vi "SS_FPGA_Drop1_all_in_v4.vi"() -> ()   [LabVIEW 2016]
uses:
  <vilib>/rvi/Emulation/niFpgaGetClockAttributes.vi
  <vilib>/rvi/Emulation/niFpgaSctlEmulationGetInTimedLoop.vi
  <vilib>/rvi/Emulation/niFpgaEmulationReportErrorSimple.vi
  <vilib>/rvi/Emulation/niFpgaCriticalErrorInLSC.vi
  <vilib>/rvi/Emulation/niFpgaProcessEmulError.vi
  <vilib>/rvi/eio/common/nirviEmuTemplateMethod_errors.vi
  <vilib>/eio/EIONode/EIONode.xnode
  <vilib>/rvi/FXPMathLib/FxpMul/XNode/nifxpmath_Multiplier.xnode
  <vilib>/rvi/FXPMathLib/FxpAdd/XNode/nifxpmath_Add.xnode
  <vilib>/rvi/FXPMathLib/sim/FxpSim.dll
panel:
  in  "Tab Control":T1(tab)
  in  "(FOR DEBUG) Overide FBIS 1kHZ":bool
  in  "Start Acquisition":bool
  out "Actual Duration (ms)":u32
  out "Number of Loop 1 Samples":i32
  in  "Scan Rate (mSec) Loop 1":u32 caption="Count(mSec)"
  in  "FSIS Interlock":bool
  out "Raw Data In Mod 1":fxp<+,24,12>[](array[numeric])
  out "Cal value out Mod 1":fxp<+,24,12>[](array[numeric]) format="%.16g"
  out "PTF - No Operations Mod 1":bool[](array[boolean])
  in  "lower limit \nNOOP mod 1":fxp<+,24,12>[](array[numeric])=[0.0, 0.0, 0.0, 0.0, 0.0, 0.0, 0.0, 0.0, 0.0, 0.0, 0.0, 0.0, 0.0, 0.0, 0.0, 0.0]
  in  "upper limit \nOKOP mod 1":fxp<+,24,12>[](array[numeric])=[0.0, 0.0, 0.0, 0.0, 0.0, 0.0, 0.0, 0.0, 0.0, 0.0, 0.0, 0.0, 0.0, 0.0, 0.0, 0.0]
  out "PTF - Warning Mod 1":bool[](array[boolean])
  in  "NOOPS Fault Filter mod 1":u16[](array[numeric])=[0, 0, 0, 0, 0, 0, 0, 0, 0, 0, 0, 0, 0, 0, 0, 0]
  in  "cal mod 1":fxp<+,24,12>[](array[numeric])=[10.0, 10.0, 10.0, 10.0, 10.0, 10.0, 10.0, 10.0, 10.0, 10.0, 10.0, 10.0, 10.0, 10.0, 10.0, 10.0]
  in  "offset mod 1":fxp<+,24,12>[](array[numeric])=[0.0, 0.0, 0.0, 0.0, 0.0, 0.0, 0.0, 0.0, 0.0, 0.0, 0.0, 0.0, 0.0, 0.0, 0.0, 0.0]
  out "Raw Data In Mod 2":fxp<+,24,12>[](array[numeric]) format="%.27g"
  in  "offset mod 2":fxp<+,24,12>[](array[numeric])=[0.0, 0.0, 0.0, 0.0, 0.0, 0.0, 0.0, 0.0, 0.0, 0.0, 0.0, 0.0, 0.0, 0.0, 0.0, 0.0]
  out "PTF - No Operations Mod 2":bool[](array[boolean])
  in  "lower limit \nNOOP mod 2":fxp<+,24,12>[](array[numeric])=[0.0, 0.0, 0.0, 0.0, 0.0, 0.0, 0.0, 0.0, 0.0, 0.0, 0.0, 0.0, 0.0, 0.0, 0.0, 0.0]
  in  "upper limit \nOKOP mod 2":fxp<+,24,12>[](array[numeric])=[0.0, 0.0, 0.0, 0.0, 0.0, 0.0, 0.0, 0.0, 0.0, 0.0, 0.0, 0.0, 0.0, 0.0, 0.0, 0.0]
  out "Cal value out Mod 2":fxp<+,24,12>[](array[numeric])
  out "PTF - Warning Mod 2":bool[](array[boolean])
  in  "NOOPS Fault Filter mod 2":u16[](array[numeric])=[0, 0, 0, 0, 0, 0, 0, 0, 0, 0, 0, 0, 0, 0, 0, 0]
  in  "cal mod 2":fxp<+,24,12>[](array[numeric])=[0.0, 0.0, 0.0, 0.0, 0.0, 0.0, 0.0, 0.0, 0.0, 0.0, 0.0, 0.0, 0.0, 0.0, 0.0, 0.0]
  out "Raw Data In Mod 3":fxp<+,24,12>[](array[numeric]) format="%.27g"
  out "PTF - No Operations Mod 3":bool[](array[boolean])
  in  "lower limit\nNOOP mod 3":fxp<+,24,12>[](array[numeric])=[0.0, 0.0, 0.0, 0.0, 0.0, 0.0, 0.0, 0.0, 0.0, 0.0, 0.0, 0.0, 0.0, 0.0, 0.0, 0.0]
  in  "upper limit\nOKOP mod 3":fxp<+,24,12>[](array[numeric])=[0.0, 0.0, 0.0, 0.0, 0.0, 0.0, 0.0, 0.0, 0.0, 0.0, 0.0, 0.0, 0.0, 0.0, 0.0, 0.0]
  out "PTF - Warning Mod 3":bool[](array[boolean])
  out "Cal value out Mod 3":fxp<+,24,12>[](array[numeric])
  in  "NOOPS Fault Filter mod 3":u16[](array[numeric])=[0, 0, 0, 0, 0, 0, 0, 0, 0, 0, 0, 0, 0, 0, 0, 0]
  in  "offset mod 3":fxp<+,24,12>[](array[numeric])=[0.0, 0.0, 0.0, 0.0, 0.0, 0.0, 0.0, 0.0, 0.0, 0.0, 0.0, 0.0, 0.0, 0.0, 0.0, 0.0]
  in  "cal mod 3":fxp<+,24,12>[](array[numeric])=[0.0, 0.0, 0.0, 0.0, 0.0, 0.0, 0.0, 0.0, 0.0, 0.0, 0.0, 0.0, 0.0, 0.0, 0.0, 0.0]
  out "Raw Data In Mod 4":fxp<+,24,12>[](array[numeric]) format="%.27g"
  out "Cal value out Mod 4":fxp<+,24,12>[](array[numeric])
  out "PTF - No Operations Mod 4":bool[](array[boolean])
  out "PTF - Warning Mod 4":bool[](array[boolean])
  in  "lower limit\nNOOP mod 4":fxp<+,24,12>[](array[numeric])=[0.0, 0.0, 0.0]
  in  "upper limit\nOKOP mod 4":fxp<+,24,12>[](array[numeric])=[0.0, 0.0, 0.0]
  in  "cal mod 4":fxp<+,24,12>[](array[numeric])=[0.0, 0.0, 0.0]
  in  "NOOPS Fault Filter mod 4":u16[](array[numeric])=[0, 0, 0]
  in  "offset mod 4":fxp<+,24,12>[](array[numeric])=[0.0, 0.0, 0.0]
  out "Cal value out Mod 5":fxp<+,24,12>[](array[numeric])
  out "PTF - No Operations Mod 5":bool[](array[boolean])
  out "PTF - Warning Mod 5":bool[](array[boolean])
  in  "lower limit\nNOOP mod 5":fxp<+,24,12>[](array[numeric])=[0.0, 0.0, 0.0]
  in  "upper limit\nOKOP mod 5":fxp<+,24,12>[](array[numeric])=[0.0, 0.0, 0.0]
  in  "cal mod 5":fxp<+,24,12>[](array[numeric])=[0.0, 0.0, 0.0]
  in  "NOOPS Fault Filter mod 5":u16[](array[numeric])=[0, 0, 0]
  in  "offset mod 5":fxp<+,24,12>[](array[numeric])=[0.0, 0.0, 0.0]
  out "Raw Data In Mod 5":fxp<+,24,12>[](array[numeric]) format="%.27g"
  out "Raw Data In Mod 6":bool[](array[boolean])
  out "Trigger from Trigger Card (SYNC and ASYNC) (Euro1Slot15)":bool
  out "Main Trigger In":bool
  out "SYNC/ASYNC":bool
  out "Beam Prepare":bool
  out "Override":bool
  out "320 Open":bool
  out "320  Closed":bool
  out "400 Open":bool
  out "400 Open Closed":bool
  out "Calorimeter Left Gate Open":bool
  out "Calorimeter Left Gate Closed":bool
  out "320  Bypass Open":bool
  out "320 Bypass Closed":bool
  out "Calorimeter Right Gate Closed":bool
  out "HV Area Water":bool
  out "MAST Area Air":bool
  out "Calorimeter Right Gate Open":bool
  # "1"
  # "2"
  # "CHANNEL ID"
  # "SS Source Body Flow\n\nSS Source Body Temperature\n\nSS Grid 1 Flow\n\nSS Grid 1 Temperature\n\nSS Grid 2 Flow\n\nSS Grid 2 Temperature\n\nSS Grid 3 Flow\n\nSS Grid 3 Temperature\n\nSS Grid 4/1st Stage Neutraliser Flow\n\nSS Grid 4/1st Stage Neutraliser Temperature\n\nSS 2nd Stage Neutraliser Flow\n\nSS 2nd Stage Neutraliser Temperature\n\nSS PINI Backplate Flow\n\nSS PINI Backplate Temperature\n\nSS Duct Scraper Flow\n\nSS Duct Scraper Temperature"
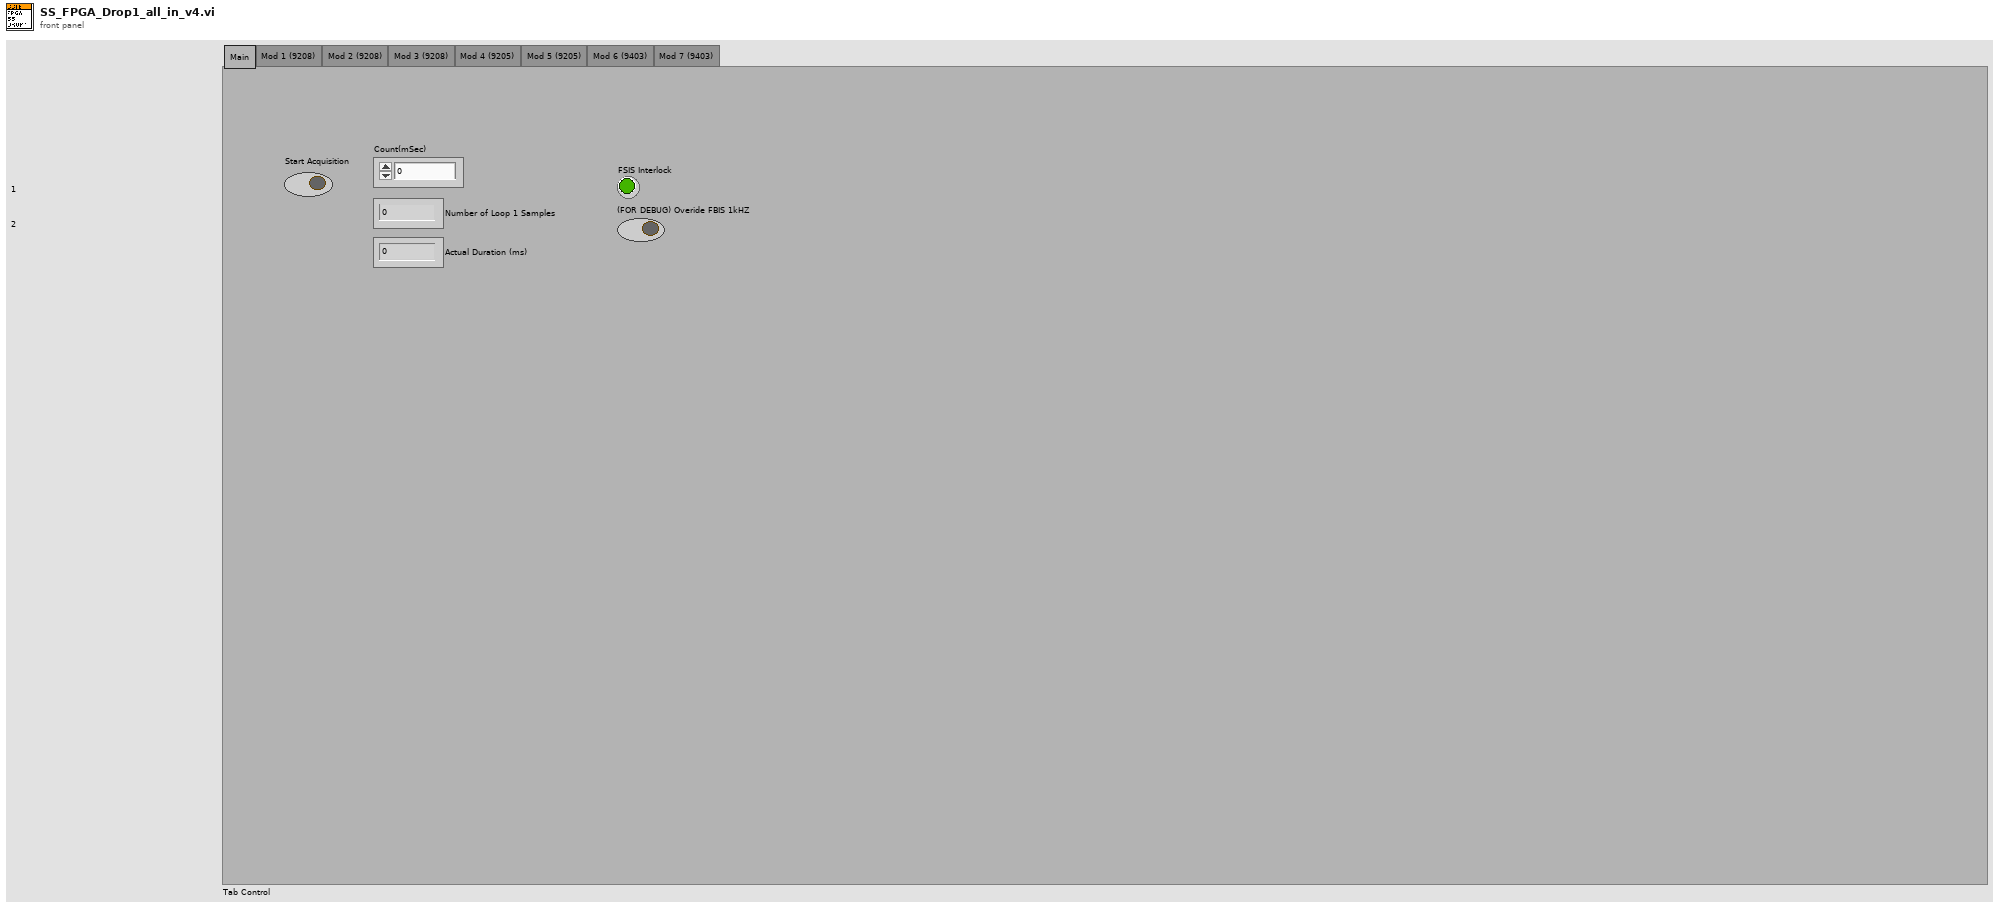
[diagram p1: front panel]
types:
  T1 = enum32{"Main", "Mod 1 (9208)", "Mod 2 (9208)", "Mod 3 (9208)", "Mod 4 (9205)", "Mod 5 (9205)", "Mod 6 (9403)", "Mod 7 (9403)"}
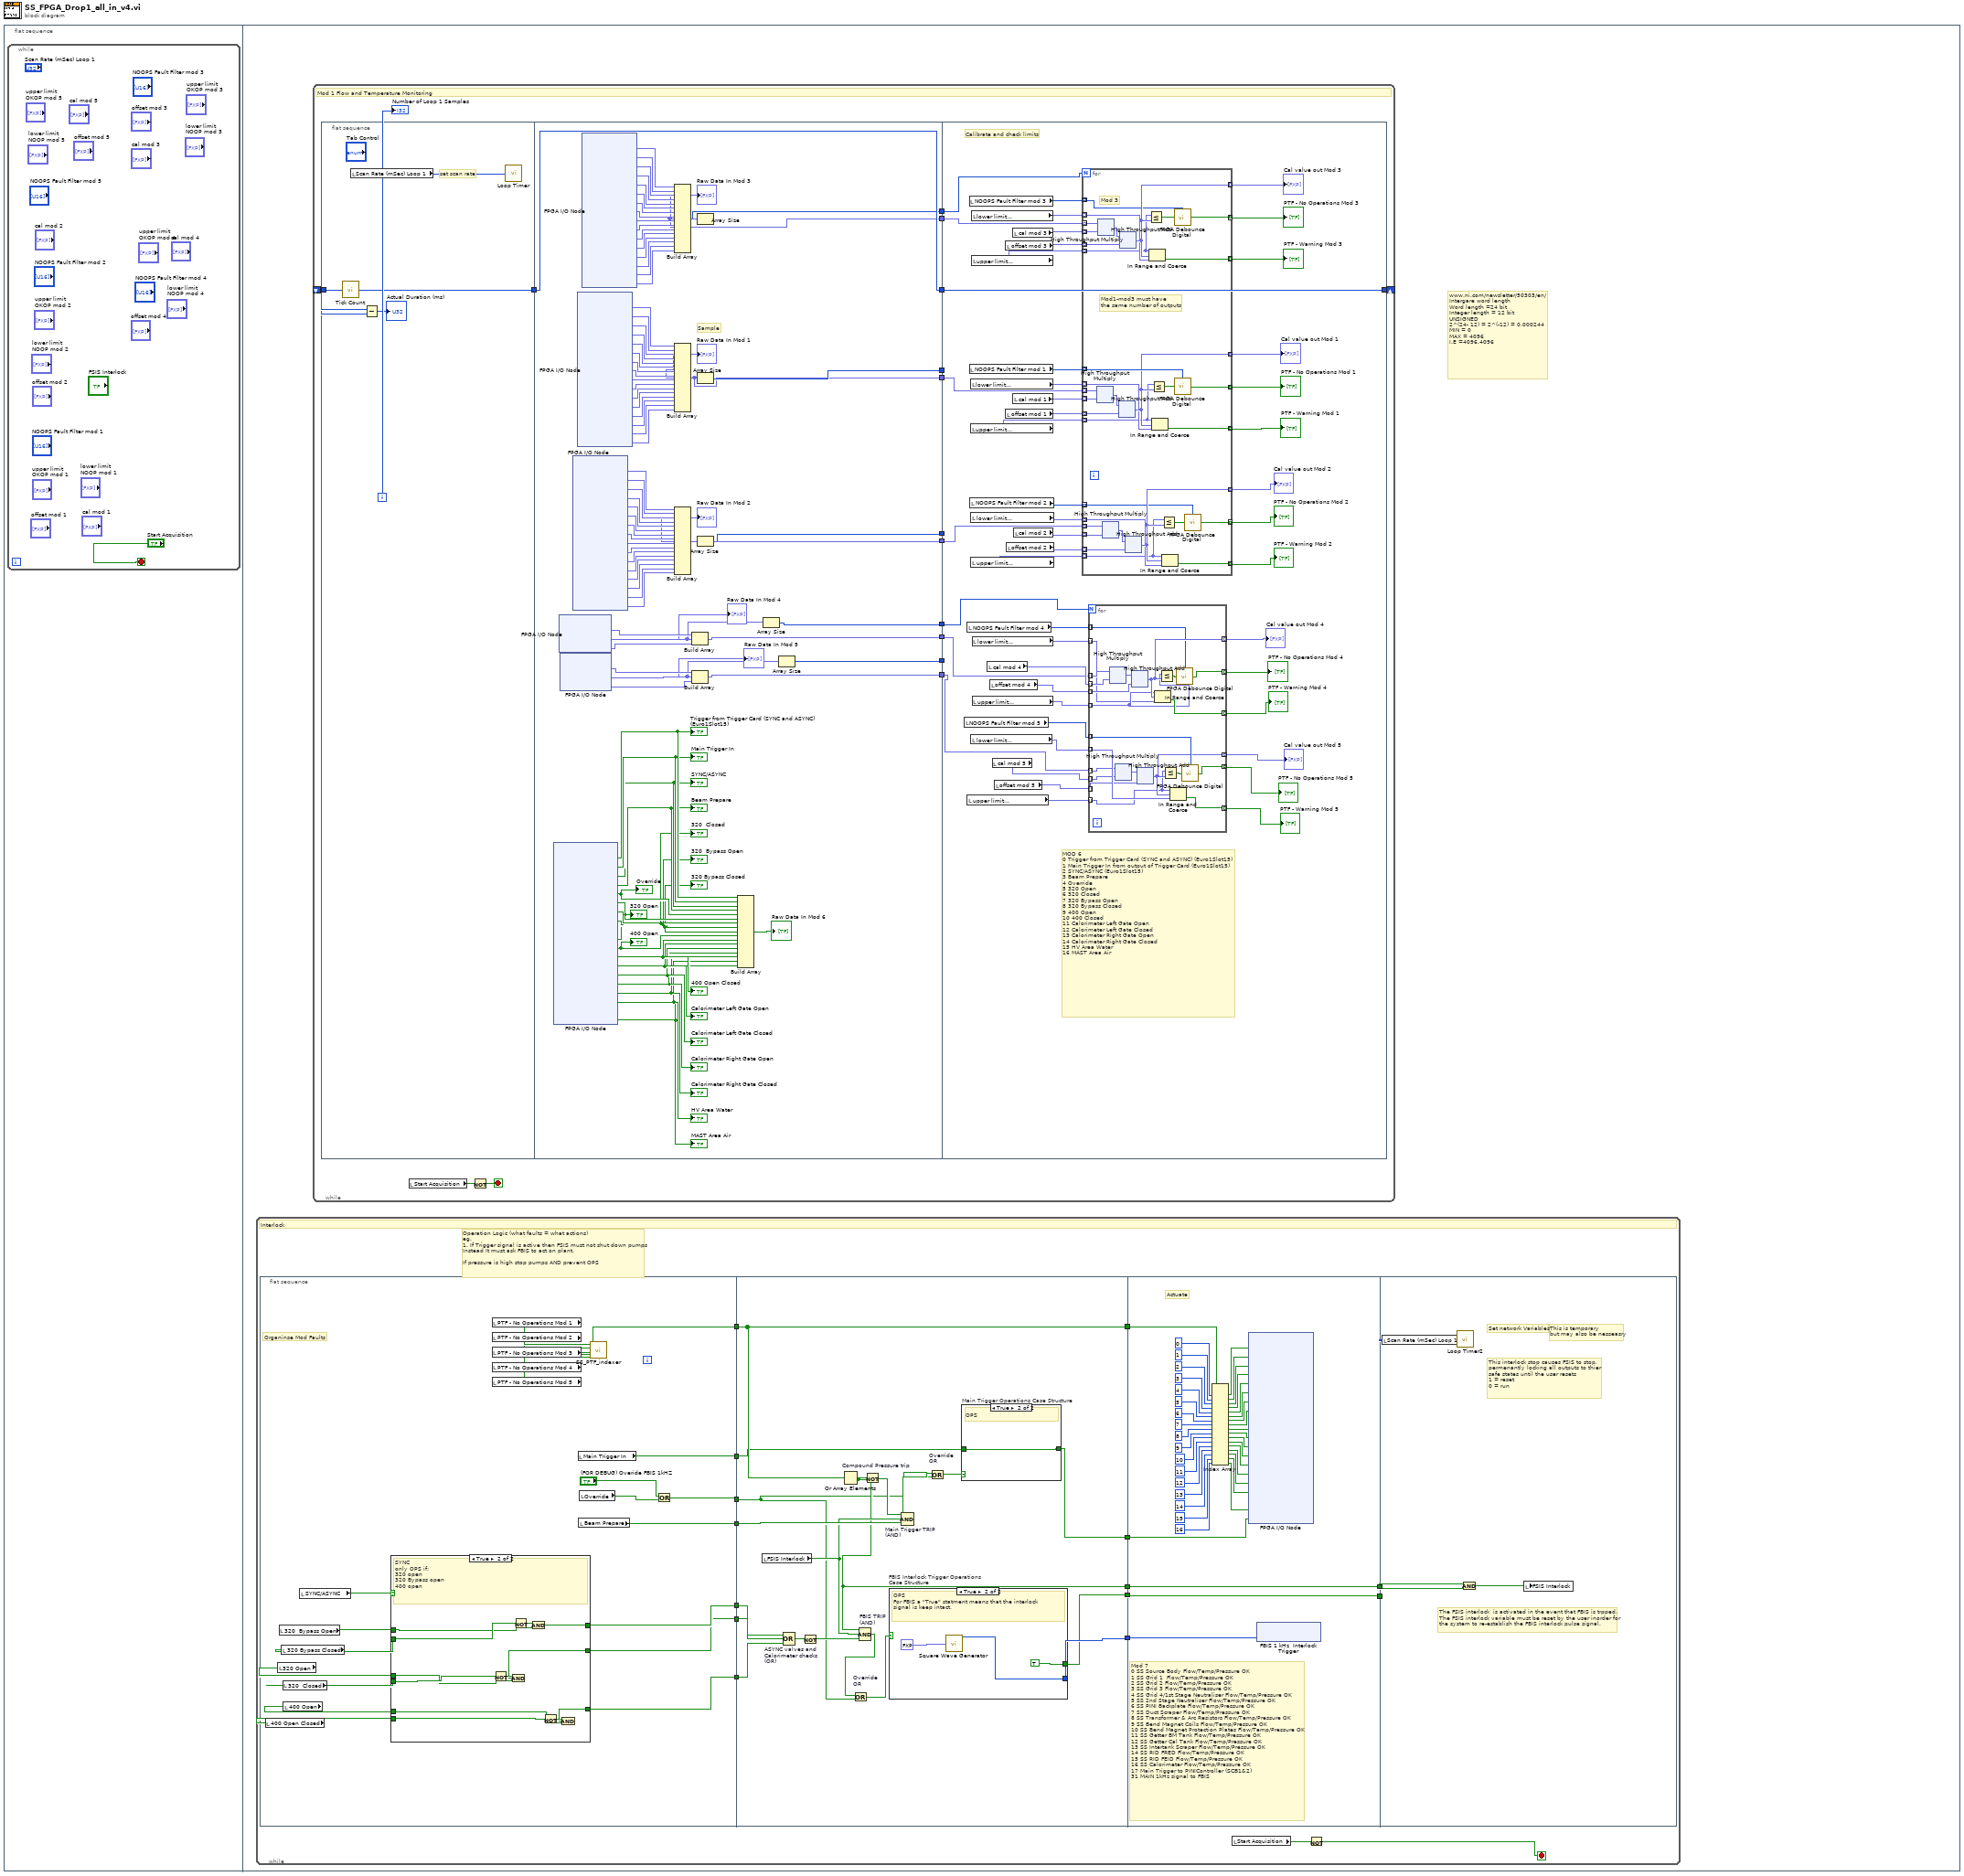
[diagram p0: block diagram]
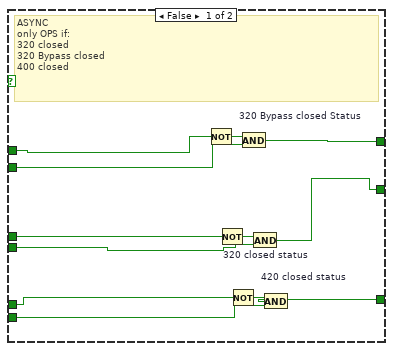
[diagram p2: hidden frame]
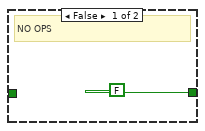
[diagram p3: hidden frame]
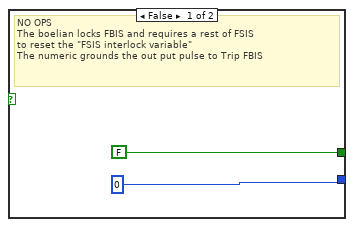
[diagram p4: hidden frame]
diagram:
  n1 = flat-sequence {
    frame #0 {
      n2 = while {
        stop <- "Start Acquisition" stop-if-true
      }
    }
    frame #1 {
      # "www.ni.com/newsletter/50303/en/\nIntergare word length \nWord length =24 bit\nInteger length = 12 bit\nUNSIGNED\n2^(24- 12) = 2^(-12) = 0.000244\nMIN = 0 \nMAX = 4096\nI.E =4096.4096"
      n3 = while {
        stop <- w8 stop-if-true
        # "Operation Logic (what faults = what actions)\neg.\n1. If Trigger signal is active then FSIS must not shut down pumps\nInstead It must ask FBIS to act on plant.\n\nIf pressure is high stop pumps AND prevent OPS"
        # "Interlock"
        n4 = flat-sequence {
          tunnel: [w32] -> w17
          tunnel: [w31] -> w16
          tunnel: [w30] -> w15
          tunnel: [w29] -> w13
          tunnel: [w24] -> w10
          tunnel: [w21] -> w3
          tunnel: [w20] -> w2
          tunnel: w17 -> [w75]
          tunnel: w16 -> [w74]
          tunnel: w15 -> [w73]
          tunnel: [w81] -> w14
          tunnel: w13 -> [w79]
          tunnel: [w68] -> w12
          tunnel: w10 -> [w80]
          tunnel: [w80] -> w9
          tunnel: [w78] -> w6
          tunnel: [w77] -> w5
          tunnel: w3 -> [w70]
          tunnel: w2 -> [w63]
          tunnel: w14 -> [w127]
          tunnel: w12 -> [w126]
          tunnel: [w126] -> w11
          tunnel: w9 -> [w125]
          tunnel: w6 -> [w90]
          tunnel: w5 -> [w89]
          tunnel: [w89] -> w4
          tunnel: w11 -> [w129]
          tunnel: w4 -> [w128]
          frame #0 {
            # "Organinse Mod Faults"
            n5 = local read "400 Open Closed"() -> (w35:bool)
            n6 = local read "320 Open"() -> (w33:bool)
            n7 = local read "320  Bypass Open"() -> (w37:bool)
            n8 = local read "320 Bypass Closed"() -> (w34:bool)
            n9 = local read "320  Closed"() -> (w22:bool)
            n10 = local read "400 Open"() -> (w36:bool)
            n11 = local read "SYNC/ASYNC"() -> (w38:bool)
            n12 = case shown="True" w38 {
              tunnel: w37 -> [w50 w58]
              tunnel: w36 -> [w42 w56]
              tunnel: w35 -> [w46 w57]
              tunnel: w34 -> [w45 w59]
              tunnel: w22 -> [w44 w55]
              tunnel: w33 -> [w43 w54]
              tunnel: [w39 w51] -> w30
              tunnel: [w41 w52] -> w31
              tunnel: [w40 w53] -> w32
              frame False {
                # "ASYNC\nonly OPS if:\n320 closed\n320 Bypass closed\n400 closed"
                n13 = Not(x=w50) -> (.not. x?=w49:bool)
                n14 = Not(x=w43) -> (.not. x?=w48:bool)
                n15 = Not(x=w42) -> (.not. x?=w47:bool)
                n16 = And "320 Bypass closed Status"(x=w49, y=w45) -> (x .and. y?=w40:bool)
                n17 = And "320 closed status"(x=w48, y=w44) -> (x .and. y?=w41:bool)
                n18 = And "420 closed status"(x=w47, y=w46) -> (x .and. y?=w39:bool)
              }
              frame True {
                # "SYNC\nonly OPS if:\n320 open\n320 Bypass open\n400 open"
                n19 = Not(x=w55) -> (.not. x?=w60:bool)
                n20 = And(x=w60, y=w54) -> (x .and. y?=w52:bool)
                n21 = Not(x=w59) -> (.not. x?=w62:bool)
                n22 = And(x=w62, y=w58) -> (x .and. y?=w53:bool)
                n23 = Not(x=w57) -> (.not. x?=w61:bool)
                n24 = And(x=w61, y=w56) -> (x .and. y?=w51:bool)
              }
            }
            n25 = local read "PTF - No Operations Mod 1"() -> (w28:bool[])
            n26 = local read "PTF - No Operations Mod 2"() -> (w27:bool[])
            n27 = local read "PTF - No Operations Mod 3"() -> (w26:bool[])
            n28 = local read "PTF - No Operations Mod 4"() -> (w25:bool[])
            n29 = local read "PTF - No Operations Mod 5"() -> (w23:bool[])
            n30 = local read "Main Trigger In"() -> (w29:bool)
            n31 = local read "Beam Prepare"() -> (w21:bool)
            n32 = local read "Override"() -> (w18:bool)
            n33 = call "SS_PTF_indexer.vi"("Faults Mod 5"=w23, "Faults Mod 4"=w25, "Faults Mod 3"=w26, "Faults Mod 2"=w27, "Faults Mod 1"=w28) -> ("Group PTF"=w24:bool[])  [unwired: 6 in]
            n34 = Or(x="(FOR DEBUG) Overide FBIS 1kHZ", y=w18) -> (x .or. y?=w20:bool)
          }
          frame #1 {
            n35 = local read "FSIS Interlock"() -> (w69:bool)
            n36 = Compound Arithmetic op=OR "ASYNC valves and \nCalorimeter checks\n(OR)"(w75, w74, w73) -> (w72:bool)
            n37 = Not(x=w72) -> (.not. x?=w71:bool)
            n38 = Or Array Elements "Compound Pressure trip"(Boolean array=w80) -> (logical OR=w76:bool)
            n39 = Not(x=w76) -> (.not. x?=w68:bool)
            n40 = Compound Arithmetic op=AND "FBIS TRIP\n(AND)"(w68, w69, w71) -> (w67:bool)
            n41 = Or "Override \nOR"(x=w67, y=w63) -> (x .or. y?=w66:bool)
            n42 = case "FBIS Interlock Trigger Operations \nCase Structure" shown="True" w66 {
              tunnel: [u8 0 ("duty cycle (periods)") w87] -> w81
              tunnel: [FALSE TRUE] -> w77
              frame False {
                # "NO OPS\nThe boelian locks FBIS and requires a rest of FSIS \nto reset the \"FSIS interlock variable\"\nThe numeric grounds the out put pulse to Trip FBIS"
              }
              frame True {
                # "OPS\nFor FBIS a \"True\" statment means that the interlock\nsignal is keep intact."
                n43 = call "Square Wave Generator"("duty cycle (periods)"=fxp<+,32,0> 0.5) -> ("square wave out"=w87:i16)  [unwired: 14 in]
              }
            }
            n44 = Compound Arithmetic op=AND "Main Trigger TRIP\n(AND)"(w68, w69, w70) -> (w64:bool)
            n45 = Or "Override \nOR"(x=w64, y=w63) -> (x .or. y?=w65:bool)
            n46 = case "Main Trigger Operations Case Structure" shown="True" w65 {
              tunnel: w79 -> [_ w83]
              tunnel: [FALSE w83] -> w78
              frame False {
                # "NO OPS"
              }
              frame True {
                # "OPS"
              }
            }
          }
          frame #2 {
            # "Mod 7\n0\tSS Source Body Flow/Temp/Pressure OK\n1\tSS Grid 1  Flow/Temp/Pressure OK\n2\tSS Grid 2 Flow/Temp/Pressure OK\n3\tSS Grid 3 Flow/Temp/Pressure OK\n4\tSS Grid 4/1st Stage Neutraliser Flow/Temp/Pressure OK\n5\tSS 2nd Stage Neutraliser Flow/Temp/Pressure OK\n6\tSS PINI Backplate Flow/Temp/Pressure OK\n7\tSS Duct Scraper Flow/Temp/Pressure OK\n8\tSS Transformer & Arc Resistors Flow/Temp/Pressure OK\n9\tSS Bend Magnet Coils Flow/Temp/Pressure OK\n10\tSS Bend Magnet Protection Plates Flow/Temp/Pressure OK\n11\tSS Getter BM Tank Flow/Temp/Pressure OK\n12\tSS Getter Cal Tank Flow/Temp/Pressure OK\n13\tSS Intertank Scraper Flow/Temp/Pressure OK\n14\tSS RID FRED Flow/Temp/Pressure OK\n15\tSS RID FEID Flow/Temp/Pressure OK\n16\tSS Calorimeter Flow/Temp/Pressure OK\n17\tMain Trigger to PINIController (SCB1&2)\n31\tMAIN 1kHz signal to FBIS"
            # "Actuate"
            n47 = Index Array(array=w125, index #1=0 ("index"), index #2=1 ("index"), index #3=2 ("index"), index #4=3 ("index"), index #5=4 ("index"), index #6=5 ("index"), index #7=6 ("index"), index #8=7 ("index"), index #9=8 ("index"), index #10=9 ("index"), index #11=10 ("index"), index #12=11 ("index"), index #13=12 ("index"), index #14=13 ("index"), index #15=14 ("index"), index #16=15 ("index"), index #17=16 ("index")) -> (element #1=w108:bool, element #2=w107:bool, element #3=w106:bool, element #4=w105:bool, element #5=w104:bool, element #6=w103:bool, element #7=w102:bool, element #8=w101:bool, element #9=w100:bool, element #10=w99:bool, element #11=w98:bool, element #12=w97:bool, element #13=w96:bool, element #14=w95:bool, element #15=w93:bool, element #16=w92:bool, element #17=w91:bool)
            n48 = xnode "FPGA I/O Node"("Mod7/DIO0"=w108, "Mod7/DIO1"=w107, "Mod7/DIO2"=w106, "Mod7/DIO3"=w105, "Mod7/DIO4"=w104, "Mod7/DIO5"=w103, "Mod7/DIO6"=w102, "Mod7/DIO7"=w101, "Mod7/DIO8"=w100, "Mod7/DIO9"=w99, "Mod7/DIO10"=w98, "Mod7/DIO11"=w97, "Mod7/DIO12"=w96, "Mod7/DIO13"=w95, "Mod7/DIO14"=w93, "Mod7/DIO15"=w92, "Mod7/DIO16"=w91, "Mod7/DIO17"=w90) -> ()  [unwired: 20 in, 22 out]
            n49 = xnode "FBIS 1 kHz  Interlock Trigger"("Mod7/DIO31:0"=w127) -> ()  [unwired: 1 in, 1 out]
          }
          frame #3 {
            # "The FSIS interlock  is activated in the event that FBIS is trpped.\nThe FSIS interlock variable must be reset by the user inorder for \nthe system to re-establish the FBIS interlock pulse signal."
            # "This interlock stop causes FSIS to stop,\npermenantly locking all outputs to thier \nsafe states until the user resets\n1 = reset\n0 = run"
            # "This is temporary\nbut may also be nesseasry"
            # "Set network Variables"
            n50 = local read "Scan Rate (mSec) Loop 1"() -> (w131:u32)
            n51 = call "Loop Timer2"("Count(mSec)"=w131) -> ()  [unwired: 1 out]
            n52 = And(x=w129, y=w128) -> (x .and. y?=w130:bool)
            n53 = local write "FSIS Interlock"(w130) -> ()
          }
        }
        n54 = local read "Start Acquisition"() -> (w7:bool)
        n55 = Not(x=w7) -> (.not. x?=w8:bool)
      }
      n56 = while {
        shift-right: [w147] -> _
        shift-left: _ -> [w145]
        i -> [w148]
        stop <- w144 stop-if-true
        # "Mod 1 Flow and Temperature Monitoring"
        n57 = flat-sequence {
          tunnel: [w149] -> w146
          tunnel: w145 -> [w150]
          tunnel: w146 -> [w219]
          tunnel: [w219] -> w142
          tunnel: [w189] -> w141
          tunnel: [w185] -> w140
          tunnel: [w184] -> w139
          tunnel: [w182] -> w138
          tunnel: [w183] -> w137
          tunnel: [w181] -> w136
          tunnel: [w173] -> w135
          tunnel: [w172] -> w134
          tunnel: [w174] -> w133
          tunnel: [w171] -> w132
          tunnel: w142 -> [w283]
          tunnel: w141 -> [_]
          tunnel: w140 -> [w272]
          tunnel: w139 -> [w282]
          tunnel: w138 -> [w277]
          tunnel: w137 -> [_]
          tunnel: w136 -> [w255]
          tunnel: [w283] -> w147
          tunnel: w135 -> [w243]
          tunnel: w134 -> [w241]
          tunnel: w133 -> [w254]
          tunnel: w132 -> [_]
          frame #0 {
            # "set scan rate"
            n58 = call "Tick Count"() -> ("Tick Count(mSec)"=w149:u32)
            n59 = local read "Scan Rate (mSec) Loop 1"() -> (w152:u32)
            n60 = Subtract(x=w149, y=w150) -> (x-y=→"Actual Duration (ms)":u32)
            n61 = call "Loop Timer"("Count(mSec)"=w152) -> ()  [unwired: 1 out]
          }
          frame #1 {
            # "Sample"
            n62 = xnode "FPGA I/O Node"() -> ("Mod6/DIO0"=w180:bool, "Mod6/DIO1"=w168:bool, "Mod6/DIO2"=w167:bool, "Mod6/DIO3"=w166:bool, "Mod6/DIO4"=w165:bool, "Mod6/DIO5"=w164:bool, "Mod6/DIO6"=w163:bool, "Mod6/DIO7"=w162:bool, "Mod6/DIO8"=w161:bool, "Mod6/DIO9"=w160:bool, "Mod6/DIO10"=w159:bool, "Mod6/DIO11"=w158:bool, "Mod6/DIO12"=w157:bool, "Mod6/DIO13"=w156:bool, "Mod6/DIO14"=w155:bool, "Mod6/DIO15"=w154:bool, "Mod6/DIO16"=w153:bool)  [unwired: 19 in, 21 out]
            "Trigger from Trigger Card (SYNC and ASYNC) (Euro1Slot15)" <- w180
            "Main Trigger In" <- w168
            "SYNC/ASYNC" <- w167
            "Beam Prepare" <- w166
            "Override" <- w165
            "320 Open" <- w164
            "320  Closed" <- w163
            "400 Open" <- w160
            "400 Open Closed" <- w159
            "Calorimeter Left Gate Open" <- w158
            "Calorimeter Left Gate Closed" <- w157
            "320  Bypass Open" <- w162
            "320 Bypass Closed" <- w161
            "Calorimeter Right Gate Closed" <- w155
            "HV Area Water" <- w154
            "MAST Area Air" <- w153
            "Calorimeter Right Gate Open" <- w156
            n63 = xnode "FPGA I/O Node"() -> ("Mod4/AI0"=w178:fxp<+/-,24,-4>, "Mod4/AI1"=w177:fxp<+/-,24,-4>, "Mod4/AI2"=w170:fxp<+/-,24,-4>)  [unwired: 3 in, 3 out]
            n64 = xnode "FPGA I/O Node"() -> ("Mod5/AI0"=w176:fxp<+/-,26,5>, "Mod5/AI1"=w175:fxp<+/-,26,5>, "Mod5/AI2"=w169:fxp<+/-,26,5>)  [unwired: 3 in, 3 out]
            n65 = xnode "FPGA I/O Node"() -> ("Mod2/AI0"=w190:fxp<+/-,24,-4>, "Mod2/AI1"=w191:fxp<+/-,24,-4>, "Mod2/AI2"=w192:fxp<+/-,24,-4>, "Mod2/AI3"=w193:fxp<+/-,24,-4>, "Mod2/AI4"=w194:fxp<+/-,24,-4>, "Mod2/AI5"=w195:fxp<+/-,24,-4>, "Mod2/AI6"=w196:fxp<+/-,24,-4>, "Mod2/AI7"=w197:fxp<+/-,24,-4>, "Mod2/AI8"=w198:fxp<+/-,24,-4>, "Mod2/AI9"=w199:fxp<+/-,24,-4>, "Mod2/AI10"=w200:fxp<+/-,24,-4>, "Mod2/AI11"=w201:fxp<+/-,24,-4>, "Mod2/AI12"=w202:fxp<+/-,24,-4>, "Mod2/AI13"=w203:fxp<+/-,24,-4>, "Mod2/AI14"=w204:fxp<+/-,24,-4>, "Mod2/AI15"=w205:fxp<+/-,24,-4>)  [unwired: 16 in, 16 out]
            n66 = xnode "FPGA I/O Node"() -> ("Mod1/AI0"=w235:fxp<+/-,24,-4>, "Mod1/AI1"=w234:fxp<+/-,24,-4>, "Mod1/AI2"=w233:fxp<+/-,24,-4>, "Mod1/AI3"=w232:fxp<+/-,24,-4>, "Mod1/AI4"=w231:fxp<+/-,24,-4>, "Mod1/AI5"=w230:fxp<+/-,24,-4>, "Mod1/AI6"=w229:fxp<+/-,24,-4>, "Mod1/AI7"=w228:fxp<+/-,24,-4>, "Mod1/AI8"=w227:fxp<+/-,24,-4>, "Mod1/AI9"=w226:fxp<+/-,24,-4>, "Mod1/AI10"=w225:fxp<+/-,24,-4>, "Mod1/AI11"=w224:fxp<+/-,24,-4>, "Mod1/AI12"=w223:fxp<+/-,24,-4>, "Mod1/AI13"=w222:fxp<+/-,24,-4>, "Mod1/AI14"=w221:fxp<+/-,24,-4>, "Mod1/AI15"=w220:fxp<+/-,24,-4>)  [unwired: 16 in, 16 out]
            n67 = xnode "FPGA I/O Node"() -> ("Mod3/AI0"=w218:fxp<+/-,24,-4>, "Mod3/AI1"=w217:fxp<+/-,24,-4>, "Mod3/AI2"=w216:fxp<+/-,24,-4>, "Mod3/AI3"=w215:fxp<+/-,24,-4>, "Mod3/AI4"=w214:fxp<+/-,24,-4>, "Mod3/AI5"=w213:fxp<+/-,24,-4>, "Mod3/AI6"=w212:fxp<+/-,24,-4>, "Mod3/AI7"=w211:fxp<+/-,24,-4>, "Mod3/AI8"=w210:fxp<+/-,24,-4>, "Mod3/AI9"=w209:fxp<+/-,24,-4>, "Mod3/AI10"=w208:fxp<+/-,24,-4>, "Mod3/AI11"=w207:fxp<+/-,24,-4>, "Mod3/AI12"=w206:fxp<+/-,24,-4>, "Mod3/AI13"=w188:fxp<+/-,24,-4>, "Mod3/AI14"=w187:fxp<+/-,24,-4>, "Mod3/AI15"=w186:fxp<+/-,24,-4>)  [unwired: 16 in, 16 out]
            n68 = Build Array(w218, w217, w216, w215, w214, w213, w212, w211, w210, w209, w208, w207, w206, w188, w187, w186) -> (w182:fxp<+/-,24,-4>[])
            "Raw Data In Mod 3" <- w182
            n69 = Build Array(w235, w234, w233, w232, w231, w230, w229, w228, w227, w226, w225, w224, w223, w222, w221, w220) -> (w185:fxp<+/-,24,-4>[])
            "Raw Data In Mod 1" <- w185
            n70 = Build Array(w190, w191, w192, w193, w194, w195, w196, w197, w198, w199, w200, w201, w202, w203, w204, w205) -> (w184:fxp<+/-,24,-4>[])
            "Raw Data In Mod 2" <- w184
            n71 = Build Array(w178, w177, w170) -> (w173:fxp<+/-,24,-4>[])
            "Raw Data In Mod 4" <- w173
            n72 = Build Array(w176, w175, w169) -> (w172:fxp<+/-,26,5>[])
            "Raw Data In Mod 5" <- w172
            n73 = Array Size(array=w182) -> (size(s)=w181:i32)
            n74 = Array Size(array=w185) -> (size(s)=w189:i32)
            n75 = Array Size(array=w184) -> (size(s)=w183:i32)
            n76 = Build Array(w180, w168, w167, w166, w165, w164, w163, w162, w161, w160, w159, w158, w157, w156, w155, w154, w153) -> (→"Raw Data In Mod 6":bool[])
            n77 = Array Size(array=w173) -> (size(s)=w174:i32)
            n78 = Array Size(array=w172) -> (size(s)=w171:i32)
          }
          frame #2 {
            # "MOD 6\n0\tTrigger from Trigger Card (SYNC and ASYNC) (Euro1Slot15)\n1\tMain Trigger In from output of Trigger Card (Euro1Slot15)\n2\tSYNC/ASYNC (Euro1Slot15)\n3\tBeam Prepare\n4\tOverride\n5\t320 Open\n6\t320 Closed\n7\t320 Bypass Open\n8\t320 Bypass Closed\n9\t400 Open \n10\t400 Closed\n11\tCalorimeter Left Gate Open\n12\tCalorimeter Left Gate Closed\n13\tCalorimeter Right Gate Open\n14\tCalorimeter Right Gate Closed\n15\tHV Area Water\n16\tMAST Area Air"
            # "Calibrate and check limits"
            n79 = local read "NOOPS Fault Filter mod 5"() -> (w236:u16[])
            n80 = local read "NOOPS Fault Filter mod 4"() -> (w247:u16[])
            n81 = local read "upper limit\nOKOP mod 5"() -> (w237:fxp<+,24,12>[])
            n82 = local read "NOOPS Fault Filter mod 3"() -> (w258:u16[])
            n83 = local read "NOOPS Fault Filter mod 1"() -> (w259:u16[])
            n84 = local read "NOOPS Fault Filter mod 2"() -> (w257:u16[])
            n85 = local read "lower limit \nNOOP mod 1"() -> (w271:fxp<+,24,12>[])
            n86 = local read "upper limit \nOKOP mod 1"() -> (w270:fxp<+,24,12>[])
            n87 = local read "lower limit \nNOOP mod 2"() -> (w278:fxp<+,24,12>[])
            n88 = local read "upper limit \nOKOP mod 2"() -> (w279:fxp<+,24,12>[])
            n89 = local read "lower limit\nNOOP mod 5"() -> (w238:fxp<+,24,12>[])
            n90 = local read "lower limit\nNOOP mod 3"() -> (w274:fxp<+,24,12>[])
            n91 = local read "upper limit\nOKOP mod 3"() -> (w273:fxp<+,24,12>[])
            n92 = local read "lower limit\nNOOP mod 4"() -> (w242:fxp<+,24,12>[])
            n93 = local read "upper limit\nOKOP mod 4"() -> (w246:fxp<+,24,12>[])
            n94 = local read "cal mod 4"() -> (w244:fxp<+,24,12>[])
            n95 = local read "offset mod 4"() -> (w245:fxp<+,24,12>[])
            n96 = local read "cal mod 5"() -> (w240:fxp<+,24,12>[])
            n97 = local read "offset mod 5"() -> (w239:fxp<+,24,12>[])
            n98 = local read "offset mod 3"() -> (w275:fxp<+,24,12>[])
            n99 = local read "offset mod 1"() -> (w268:fxp<+,24,12>[])
            n100 = local read "offset mod 2"() -> (w281:fxp<+,24,12>[])
            n101 = local read "cal mod 3"() -> (w276:fxp<+,24,12>[])
            n102 = local read "cal mod 1"() -> (w269:fxp<+,24,12>[])
            n103 = local read "cal mod 2"() -> (w280:fxp<+,24,12>[])
            n104 = for {
              N: w255 -> [_]
              tunnel: w282 -> [w338] mode=indexing
              tunnel: w281 -> [w337] mode=indexing
              tunnel: w280 -> [w336] mode=indexing
              tunnel: w279 -> [w308] mode=indexing
              tunnel: w278 -> [w311] mode=indexing
              tunnel: w277 -> [w335] mode=indexing
              tunnel: w276 -> [w334] mode=indexing
              tunnel: w275 -> [w333] mode=indexing
              tunnel: w274 -> [w309] mode=indexing
              tunnel: w273 -> [w306] mode=indexing
              tunnel: w272 -> [w332] mode=indexing
              tunnel: w271 -> [w310] mode=indexing
              tunnel: w270 -> [w307] mode=indexing
              tunnel: w269 -> [w331] mode=indexing
              tunnel: w268 -> [w330] mode=indexing
              tunnel: [w329] -> w267 mode=indexing
              tunnel: [w328] -> w266 mode=indexing
              tunnel: [w327] -> w265 mode=indexing
              tunnel: [w326] -> w264 mode=indexing
              tunnel: [w325] -> w263 mode=indexing
              tunnel: [w324] -> w262 mode=indexing
              tunnel: [w323] -> w261 mode=indexing
              tunnel: [w322] -> w260 mode=indexing
              tunnel: w259 -> [w321] mode=indexing
              tunnel: w258 -> [w320] mode=indexing
              tunnel: w257 -> [w319] mode=indexing
              tunnel: [w318] -> w256 mode=indexing
              # "Mod1-mod3 must have \nthe same number of outputs"
              # "Mod 3"
              n105 = xnode ("High Throughput Multiply")("x"=w332, "y"=w331) -> ("x*y"=w314:fxp<+,24,12>)
              n106 = xnode ("High Throughput Multiply")("x"=w335, "y"=w334) -> ("x*y"=w316:fxp<+,24,12>)
              n107 = xnode ("High Throughput Multiply")("x"=w338, "y"=w336) -> ("x*y"=w312:fxp<+,24,12>)
              n108 = xnode ("High Throughput Add")("x"=w314, "y"=w330) -> ("x+y"=w318:fxp<+,24,12>)
              n109 = xnode ("High Throughput Add")("x"=w316, "y"=w333) -> ("x+y"=w329:fxp<+,24,12>)
              n110 = xnode ("High Throughput Add")("x"=w312, "y"=w337) -> ("x+y"=w328:fxp<+,24,12>)
              n111 = Less Or Equal?(x=w306, y=w329) -> (x <= y?=w317:bool)
              n112 = In Range and Coerce(upper limit=w306, x=w329, lower limit=w309) -> (In Range?=w327:bool)  [unwired: 1 out]
              n113 = Less Or Equal?(x=w307, y=w318) -> (x <= y?=w315:bool)
              n114 = In Range and Coerce(upper limit=w307, x=w318, lower limit=w310) -> (In Range?=w324:bool)  [unwired: 1 out]
              n115 = Less Or Equal?(x=w308, y=w328) -> (x <= y?=w313:bool)
              n116 = In Range and Coerce(upper limit=w308, x=w328, lower limit=w311) -> (In Range?=w322:bool)  [unwired: 1 out]
              n117 = call "FPGA Debounce Digital.vi"("Input Signal"=w317, "Cycles to Filter"=w320) -> ("Output Filtered Signal"=w326:bool)
              n118 = call "FPGA Debounce Digital.vi"("Input Signal"=w315, "Cycles to Filter"=w321) -> ("Output Filtered Signal"=w325:bool)
              n119 = call "FPGA Debounce Digital.vi"("Input Signal"=w313, "Cycles to Filter"=w319) -> ("Output Filtered Signal"=w323:bool)
            }
            "Cal value out Mod 1" <- w256
            "Cal value out Mod 3" <- w267
            "Cal value out Mod 2" <- w266
            "PTF - No Operations Mod 1" <- w263
            "PTF - Warning Mod 1" <- w262
            "PTF - No Operations Mod 3" <- w264
            "PTF - Warning Mod 3" <- w265
            "PTF - No Operations Mod 2" <- w261
            "PTF - Warning Mod 2" <- w260
            n120 = for {
              N: w254 -> [_]
              tunnel: [w289] -> w253 mode=indexing
              tunnel: [w288] -> w252 mode=indexing
              tunnel: [w287] -> w251 mode=indexing
              tunnel: [w303] -> w250 mode=indexing
              tunnel: [w302] -> w249 mode=indexing
              tunnel: [w301] -> w248 mode=indexing
              tunnel: w247 -> [w300] mode=indexing
              tunnel: w246 -> [w286] mode=indexing
              tunnel: w245 -> [w299] mode=indexing
              tunnel: w244 -> [w298] mode=indexing
              tunnel: w243 -> [w297] mode=indexing
              tunnel: w242 -> [w285] mode=indexing
              tunnel: w241 -> [w292] mode=indexing
              tunnel: w240 -> [w291] mode=indexing
              tunnel: w239 -> [w290] mode=indexing
              tunnel: w238 -> [w293] mode=indexing
              tunnel: w237 -> [w284] mode=indexing
              tunnel: w236 -> [w294] mode=indexing
              n121 = xnode ("High Throughput Multiply")("x"=w297, "y"=w298) -> ("x*y"=w304:fxp<+,24,12>)
              n122 = xnode ("High Throughput Multiply")("x"=w292, "y"=w291) -> ("x*y"=w295:fxp<+,24,12>)
              n123 = xnode ("High Throughput Add")("x"=w304, "y"=w299) -> ("x+y"=w303:fxp<+,24,12>)
              n124 = xnode ("High Throughput Add")("x"=w295, "y"=w290) -> ("x+y"=w287:fxp<+,24,12>)
              n125 = In Range and Coerce(upper limit=w286, x=w303, lower limit=w285) -> (In Range?=w301:bool)  [unwired: 1 out]
              n126 = Less Or Equal?(x=w286, y=w303) -> (x <= y?=w305:bool)
              n127 = Less Or Equal?(x=w284, y=w287) -> (x <= y?=w296:bool)
              n128 = In Range and Coerce(upper limit=w284, x=w287, lower limit=w293) -> (In Range?=w289:bool)  [unwired: 1 out]
              n129 = call "FPGA Debounce Digital.vi"("Input Signal"=w305, "Cycles to Filter"=w300) -> ("Output Filtered Signal"=w302:bool)
              n130 = call "FPGA Debounce Digital.vi"("Input Signal"=w296, "Cycles to Filter"=w294) -> ("Output Filtered Signal"=w288:bool)
            }
            "Cal value out Mod 4" <- w250
            "PTF - No Operations Mod 4" <- w249
            "PTF - Warning Mod 4" <- w248
            "PTF - Warning Mod 5" <- w253
            "Cal value out Mod 5" <- w251
            "PTF - No Operations Mod 5" <- w252
          }
        }
        n131 = local read "Start Acquisition"() -> (w143:bool)
        n132 = Not(x=w143) -> (.not. x?=w144:bool)
        "Number of Loop 1 Samples" <- w148
      }
    }
  }
